vi "test_poisson.vi"() -> ()   [LabVIEW 2010]
uses:
  <vilib>/gmath/statdist.llb/Poisson CDF.vi
  <vilib>/gmath/statdist.llb/Poisson Inverse CDF.vi
  <vilib>/gmath/NI_Gmath.lvlib
panel:
  out "k":i32
  out "F(X=k) =prob (X<=k)":dbl=0.7357588823428847
  in  "F(k)":dbl caption="F(X=k)"
  in  "m":dbl=1.0
  in  "k":dbl=1.0 caption="X=k"
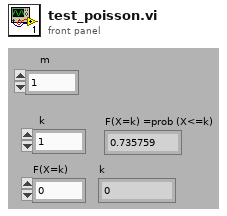
[diagram p1: front panel]
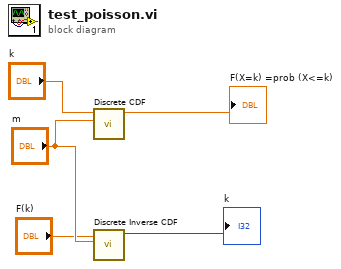
[diagram p0: block diagram]
diagram:
  n1 = call-poly <vilib>:"Discrete CDF.vi"("lambda"="m", "x"="k") -> ("cdf(x)"=→"F(X=k) =prob (X<=k)":dbl)  [unwired: 8 in, 1 out]
  n2 = call-poly <vilib>:"Discrete Inverse CDF.vi"("lambda"="m", "cdf(x)"="F(k)") -> ("x"=→"k":i32)  [unwired: 8 in, 1 out]
